vi "BonOMM-SAOMM.vi"() -> ()   [LabVIEW 2019] (continued)
                                n1114 = Insert Into Array(array=w4646, index=5, new element=w4645) -> (w4643:string[])
                                }
                                n1115 = local write "loaded_lib"(w4636) -> ()
                                n1116 = local write "Librairie des objets"(w4637) -> ()
                                n1117 = local write "Librairie complète"(w4637) -> ()
                              }
                            }
                          }
                          frame True {
                          }
                        }
                      }
                      frame "scp_Charger une libraire d'objets" {
                        # "Chemin à confirmer,\nvoir avec Mr Turbide ..."
                        # "Gestion du menu en développement ..."
                        n1118 = local read "path_libdir"() -> (w4657:path)
                        n1119 = File Dialog(6:"*.txt" ("pattern"), 7:"Sélectionner la libraire désirée ..." ("prompt"), 11:w4657) -> (0:w4658:errorcluster, 2:w4662:bool, 3:w4659:path)  [unwired: 4 in, 1 out]
                        n1120 = Unbundle(w4658) -> ()  [unwired: 3 out]
                        n1121 = case shown="Vrai" w4662 {
                          tunnel: w4659 -> [_ w4668]
                          frame False {
                          }
                          frame True {
                            n1122 = local write "loaded_lib"(w4668) -> ()
                            n1123 = local read "LST"() -> (w4665:dbl)
                            n1124 = call "Read_obs_files.vi"("Path"=w4668) -> ("Output Table"=w4673:string[][])  [unwired: 1 out]
                            n1125 = Strip Path(path=w4668) -> (stripped path=w4667:path)  [unwired: 1 out]
                            n1126 = for {
                              tunnel: w4673 -> [w4679] mode=indexing
                              tunnel: w4665 -> [w4680]
                              tunnel: [w4676] -> w4664 mode=indexing
                              n1127 = Index Array(array=w4679, index #1=2 ("index"), index #2=3 ("index")) -> (element #1=w4682:string, element #2=w4681:string)
                              n1128 = call "Airmass.vi"("temps sidéral"=w4680, "DEC"=w4681, "RA"=w4682) -> ("airmass"=w4677:dbl)
                              n1129 = Number To Fractional String(number=w4677, precision (6)=i16 2) -> (F-format string=w4678:string)  [unwired: 2 in]
                              n1130 = Insert Into Array(array=w4679, index=5, new element=w4678) -> (w4676:string[])
                            }
                            n1131 = Path To String(path=w4667) -> (string=w4669:string)
                            n1132 = local write "Librairie des objets"(w4664) -> ()
                            n1133 = control-ref of="TERMINAL"() -> (w4666:refnum<vi>)
                            n1134 = control-ref of="Indicateur d'état"() -> (w4663:refnum<vi>)
                            n1135 = Concatenate Strings("Chargement de la librairie \"", w4669, "\"") -> (w4672:string)
                            n1136 = call "TERMINAL.vi"("Indicateur Refnum"=w4663, "Terminal Refnum"=w4666, "Indicateur d'état"=w4672) -> ()
                          }
                        }
                      }
                      frame "scp_Modifier la liste des filtres" {
                        n1137 = call "ChoixFiltres.vi"("Ordre des filtres Avant"="Tableau des filtres") -> ("Ordre des filtres Après"=w4685:string[])
                        n1138 = local write "Tableau des filtres"(w4685) -> ()
                      }
                      frame "scp_Calibration du foyer automatique" {
                        # "À refaire avec le nouveau détecteur ..."
                      }
                      frame "scp_Calibration du champ" {
                        n1139 = local read "CentreTel X"() -> (w4690:dbl)
                        n1140 = local read "CentreTel Y"() -> (w4689:dbl)
                        n1141 = local read "Reference X"() -> (w4688:dbl)
                        n1142 = local read "Reference Y"() -> (w4687:dbl)
                        n1143 = local read "TableAstrom"() -> (w4692:T4)
                        n1144 = call "Starast.vi"("Ry"=w4687, "Rx"=w4688, "Centre Y"=w4689, "Centre X"=w4690, "Table Astrometry IN"=w4692) -> ("Table Astrometry OUT"=w4691:T4)  [unwired: 6 in]
                        n1145 = local write "TableAstrom"(w4691) -> ()
                      }
                    }
                  }
                  frame "main_Télescope" {
                    n1146 = case shown="\"tel_Test signal vers TCS\"" w4693 {
                      frame Default {
                      }
                      frame "tel_Synchroniser la coupole" {
                        n1147 = stacked-sequence {
                          frame #0 {
                            n1148 = control-ref of="TERMINAL"() -> (w4696:refnum<vi>)
                            n1149 = control-ref of="Indicateur d'état"() -> (w4695:refnum<vi>)
                            n1150 = call "TERMINAL.vi"("Indicateur Refnum"=w4695, "Terminal Refnum"=w4696, "Indicateur d'état"="Synchronisation de la coupole sur la position du télescope") -> ()
                          }
                          frame #1 {
                            # "Synchronise la coupole a la \nposition du télescope"
                            n1151 = control-ref of="TCS actif"() -> (w4697:refnum<vi>)
                            n1152 = local read "TCS VRN"() -> (w4704:refnum<visa-resource-name>)
                            n1153 = Build Array(0.0 ("string1")) -> (w4702:dbl[])
                            n1154 = call "EXCOM-CMD.vi"("VRN IN"=w4704, "Bool Refnum"=w4697, "Commande #"=2, "Args"=w4702) -> ("VRN OUT"=w4700:refnum<visa-resource-name>, "OK Done"=w4699:bool, "Error OUT"=w4698:errorcluster)  [unwired: 9 in]
                            n1155 = local write "TCS Error"(w4698) -> ()
                            n1156 = local write "TCS VRN"(w4700) -> ()
                            n1157 = case shown="Faux" w4699 {
                              frame False {
                                n1158 = One Button Dialog(message="ATTENTION!!\nLa commande de synchronisation de la coupole a échouée.\nVérifiez la communication avec TCS et recommencez.", button name ("OK")="OK" ("nom du bouton (\"OK\")")) -> ()  [unwired: 1 out]
                              }
                              frame True {
                              }
                            }
                          }
                        }
                      }
                      frame "tel_Synchroniser les horloges" {
                        n1159 = stacked-sequence {
                          seq-local: [w4710 _ _ _] -> [_ _ _ w4728]
                          frame #0 {
                            n1160 = local read "Epoch Tel"() -> (w4710:dbl)
                          }
                          frame #1 {
                            # "Initialise TCS"
                            n1161 = call "GetUTC.vi"() -> ("UTC_fractional"=w4720:dbl, "Day"=w4719:dbl, "Month"=w4718:dbl, "Year"=w4717:dbl, "DST?"=→"DST?":bool)  [unwired: 4 out]
                            n1162 = control-ref of="TCS actif"() -> (w4711:refnum<vi>)
                            n1163 = local read "TCS VRN"() -> (w4722:refnum<visa-resource-name>)
                            n1164 = Build Array(w4717, w4718, w4719, w4720) -> (w4716:dbl[])
                            n1165 = call "EXCOM-CMD.vi"("VRN IN"=w4722, "Bool Refnum"=w4711, "Commande #"=1, "Args"=w4716) -> ("VRN OUT"=w4715:refnum<visa-resource-name>, "OK Done"=w4714:bool, "Error OUT"=w4713:errorcluster)  [unwired: 9 in]
                            n1166 = local write "TCS Error"(w4713) -> ()
                            n1167 = local write "TCS VRN"(w4715) -> ()
                            n1168 = case shown="Vrai" w4714 {
                              frame False {
                                n1169 = One Button Dialog(message="ATTENTION!!\nLa commande INITIALISE TCS\na échoué.\nVérifiez TCS.", button name ("OK")="OK" ("nom du bouton (\"OK\")")) -> ()  [unwired: 1 out]
                              }
                              frame True {
                                n1170 = Wait (ms)(milliseconds to wait=u32 10 ("attente (ms)")) -> ()  [unwired: 1 out]
                              }
                            }
                          }
                          frame #2 {
                            n1171 = Wait (ms)(milliseconds to wait=u32 250) -> ()  [unwired: 1 out]
                          }
                          frame #3 {
                            n1172 = control-ref of="TCS actif"() -> (w4727:refnum<vi>)
                            n1173 = local read "TCS VRN"() -> (w4730:refnum<visa-resource-name>)
                            n1174 = Build Array(w4728) -> (w4733:dbl[])
                            n1175 = call "EXCOM-CMD.vi"("VRN IN"=w4730, "Bool Refnum"=w4727, "Commande #"=22, "Args"=w4733) -> ("VRN OUT"=w4731:refnum<visa-resource-name>, "Error OUT"=w4729:errorcluster)  [unwired: 9 in, 1 out]
                            n1176 = local write "TCS VRN"(w4731) -> ()
                            n1177 = local write "TCS Error"(w4729) -> ()
                          }
                        }
                        n1178 = control-ref of="TERMINAL"() -> (w4709:refnum<vi>)
                        n1179 = control-ref of="Indicateur d'état"() -> (w4708:refnum<vi>)
                        n1180 = call "TERMINAL.vi"("Indicateur Refnum"=w4708, "Terminal Refnum"=w4709, "Indicateur d'état"="Commande d'initialisation de TCS") -> ()
                      }
                      frame "tel_Modifier la vitesse du télescope" {
                        # "Changer la vitesse"
                        n1181 = control-ref of="TCS actif"() -> (w4734:refnum<vi>)
                        n1182 = local read "TCS VRN"() -> (w4738:refnum<visa-resource-name>)
                        n1183 = local read "TCS Error"() -> (w4736:errorcluster)
                        n1184 = control-ref of="TERMINAL"() -> (w4741:refnum<vi>)
                        n1185 = control-ref of="Indicateur d'état"() -> (w4742:refnum<vi>)
                        n1186 = call "Set speed.vi"("VRN IN"=w4738, "Bool Refnum"=w4734, "error IN"=w4736) -> ("VRN OUT"=w4737:refnum<visa-resource-name>, "OK Done"=w4739:bool, "error out"=w4735:errorcluster)  [unwired: 10 in]
                        n1187 = local write "TCS VRN"(w4737) -> ()
                        n1188 = local write "TCS Error"(w4735) -> ()
                        n1189 = call "TERMINAL.vi"("Indicateur Refnum"=w4742, "Terminal Refnum"=w4741, "Indicateur d'état"="Commande de changement des vitesse de TCS") -> ()
                        n1190 = case shown="Faux" w4739 {
                          frame False {
                            n1191 = One Button Dialog(message="ATTENTION!!\nLa commande CHANGER VITESSE a échoué.\nVérifiez TCS.", button name ("OK")="OK" ("nom du bouton (\"OK\")")) -> ()  [unwired: 1 out]
                          }
                          frame True {
                          }
                        }
                      }
                      frame "tel_Modifier la vitesse de guidage" {
                        n1192 = local read "RateRA"() -> (w4749:dbl)
                        n1193 = expression code="1000/x"(w4749) -> (w4748:dbl)
                        n1194 = call "GuideRate.vi"("Guide Rate"=w4748) -> ("Guide Rate out"=w4746:dbl)  [unwired: 14 in]
                        n1195 = Build Array(w4746) -> (w4747:dbl[])
                        n1196 = expression code="1000/x"(w4746) -> (w4745:dbl)
                        n1197 = control-ref of="TCS actif"() -> (w4752:refnum<vi>)
                        n1198 = local read "TCS VRN"() -> (w4753:refnum<visa-resource-name>)
                        n1199 = call "EXCOM-CMD.vi"("VRN IN"=w4753, "Bool Refnum"=w4752, "Commande #"=15, "Args"=w4747) -> ("VRN OUT"=w4754:refnum<visa-resource-name>, "Error OUT"=w4750:errorcluster)  [unwired: 9 in, 1 out]
                        n1200 = local write "RateDEC"(w4745) -> ()
                        n1201 = local write "RateRA"(w4745) -> ()
                        n1202 = local write "TCS Error"(w4750) -> ()
                        n1203 = local write "TCS VRN"(w4754) -> ()
                      }
                      frame "tel_Modifier l'époque d'affichage" {
                        # "Ne change pas l'équinoxe de TCS mais seulement l'affichage pour BonOMM"
                        n1204 = local read "Epoch Tel"() -> (w4756:dbl)
                        n1205 = local read "AnnéeRL"() -> (w4757:dbl)
                        n1206 = call "Set_epoch.vi"("AnnéeRL"=w4757, "EPOCH_AFF"=w4756) -> ("EPOCH_OUT"=w4755:dbl)
                        n1207 = local write "dflt-EQX"(w4755) -> ()
                        n1208 = disable-structure shown="Disabled" {
                          disable-tunnel: w4755 -> [w4758 _]
                          frame Disabled {
                            n1209 = control-ref of="TCS actif"() -> (w4759:refnum<vi>)
                            n1210 = local read "TCS VRN"() -> (w4765:refnum<visa-resource-name>)
                            n1211 = Build Array(w4758) -> (w4760:dbl[])
                            n1212 = call "EXCOM-CMD.vi"("VRN IN"=w4765, "Bool Refnum"=w4759, "Commande #"=22 ("NombredArguments"), "Args"=w4760) -> ("VRN OUT"=w4763:refnum<visa-resource-name>, "OK Done"=w4761:bool, "Error OUT"=w4762:errorcluster)  [unwired: 9 in]
                            n1213 = local write "TCS Error"(w4762) -> ()
                            n1214 = local write "TCS VRN"(w4763) -> ()
                            n1215 = case shown="Faux" w4761 {
                              frame False {
                                n1216 = One Button Dialog(message="Erreur lors du chargement de la nouvelle époque d'affichage.\nVérifier la communication avec TCS et recommencez.") -> ()  [unwired: 1 in, 1 out]
                              }
                              frame True {
                              }
                            }
                          }
                          frame Enabled {
                          }
                        }
                      }
                      frame "tel_Test signal vers TCS" {
                        n1217 = call "Test_telecommande.vi"() -> ()  [unwired: 1 in]
                      }
                      frame "tel_Reconnexion" {
                        n1218 = One Button Dialog(message="Devrait reconnecter TCS ...") -> ()  [unwired: 1 in, 1 out]
                      }
                    }
                  }
                  frame "main_Secondaire Actif" {
                    n1219 = case shown="\"hex_Déplacement manuel\"" w4768 {
                      frame Default {
                      }
                      frame "hex_Commander l'hexapode" {
                        n1220 = flat-sequence {
                          frame #0 {
                            "HexaSpam" <- TRUE ("HexaSpam")
                          }
                          frame #1 {
                            # "Attention, erreur d'époque possible ..."
                            n1221 = disable-structure shown="Disabled" {
                              frame Disabled {
                                # "Rafraichi la position de l'hexapode 2x par seconde"
                                n1222 = local read "Hexapod VRN"() -> (w4786:refnum<visa-resource-name>)
                                n1223 = local read "MessageType"() -> (w4787:cluster{string[], u32[]})
                                n1224 = local read "PrAMS VRN"() -> (w4789:refnum<visa-resource-name>)
                                n1225 = control-ref of="HexX"() -> (w4772:refnum<vi>)
                                n1226 = control-ref of="HexY"() -> (w4773:refnum<vi>)
                                n1227 = control-ref of="HexZ"() -> (w4774:refnum<vi>)
                                n1228 = control-ref of="HexU"() -> (w4775:refnum<vi>)
                                n1229 = control-ref of="HexV"() -> (w4776:refnum<vi>)
                                n1230 = local read "Signature"() -> (w4788:u32)
                                n1231 = Bundle("PrAMS VRN"=w4789, "Signature"=w4788, "MessageType"=w4787, "Hexapod VRN"=w4786) -> (w4785:T28)  [unwired: 1 in]
                                n1232 = Bundle("HexX"=w4772, "HexY"=w4773, "HexZ"=w4774, "HexU"=w4775, "HexV"=w4776) -> (w4771:T29)  [unwired: 1 in]
                                n1233 = control-ref of="Angle Hor."() -> (w4779:refnum<vi>)
                                n1234 = control-ref of="DEC Tel"() -> (w4778:refnum<vi>)
                                n1235 = control-ref of="PrAMS-ACK"() -> (w4781:refnum<vi>)
                                n1236 = control-ref of="Hexapod-ACK"() -> (w4783:refnum<vi>)
                                n1237 = control-ref of="Epoch Tel"() -> (w4770:refnum<vi>)
                                n1238 = control-ref of="PrAMS actif"() -> (w4784:refnum<vi>)
                                n1239 = control-ref of="HexaCons actif"() -> (w4782:refnum<vi>)
                                n1240 = Bundle("Angle Hor."=w4779, "DEC Tel"=w4778, "Epoch Tel"=w4770) -> (w4777:T30)  [unwired: 1 in]
                                n1241 = flat-sequence {
                                tunnel: w4785 -> [w4793]
                                tunnel: w4780 -> [w4792]
                                tunnel: w4777 -> [w4791]
                                tunnel: w4771 -> [w4790]
                                frame #0 {
                                n1242 = call "Hexapod-Console.vi"("CommCluster"=w4793, "ReferenceCluster"=w4792, "TelescopeCLuster"=w4791, "HexapodCluster"=w4790) -> ()  [unwired: 12 in]
                                }
                                frame #1 {
                                n1243 = local write "HexaSpam"(FALSE ("HexaSpam")) -> ()
                                }
                                }
                                n1244 = while {
                                stop <- w4796 continue-if-true
                                n1245 = Wait (ms)(milliseconds to wait=u32 500) -> ()  [unwired: 1 out]
                                n1246 = local read "HexaSpam"() -> (w4796:bool)
                                n1247 = property on="HexapodRefresh" class="Bool (strict)"("Val(Sgnl)"=TRUE ("Value (Signaling)")) -> ()  [unwired: 2 in, 2 out]
                                }
                                n1248 = Bundle("PrAMS actif"=w4784, "PrAMS-ACK"=w4781, "HexaCons actif"=w4782, "Hexapod-ACK"=w4783) -> (w4780:T31)  [unwired: 1 in]
                              }
                              frame Enabled {
                                n1249 = One Button Dialog(message="Fonction en développement ...\n\nUtilisez plutôt \"déplacement manuel\"") -> ()  [unwired: 1 in, 1 out]
                              }
                            }
                          }
                        }
                      }
                      frame "hex_Paramètres d'asservissement" {
                        # "Ici, on voudra probablement :\n  - Modifier la fréquence du filtre\n  - Modifier le nombre d'image prises en compte\n  - Modifier le coefficient d'aggressivité\n  - Modifier l'affichage de l'historique"
                        n1250 = One Button Dialog(message="Interaction usagé à définir ...") -> ()  [unwired: 1 in, 1 out]
                      }
                      frame "hex_Panneau de offset" {
                        n1251 = flat-sequence {
                          tunnel: [w4806] -> w4800
                          tunnel: w4800 -> [w4813]
                          frame #0 {
                            n1252 = local read "Mode"() -> (w4801:u16)
                            n1253 = case shown="0" w4801 {
                              frame Default {
                              }
                              frame 0 {
                                n1254 = One Button Dialog(message="Il semble que le système ne soit pas en mode \"collimation\".\n\nPour que les valeurs de offsets demandés prennent effets, il\nest essentiel que le système soit en mode \"collimation\" ou \ntout autre mode utilisant l'hexapode.\n\nPour lancer le mode collimation, lancer d'abord l'exposition\nde la caméra de guidage puis sélectionné \"collimation\".\n\nL'application permettant de charger les offsets d'hexapode\nsera tout de même lancé, mais l'effet ne sera appliqué que\nlors du lancement d'un des modes utilisant l'hexapode.", button name ("OK")="J'ai lu et compris, merci.") -> ()  [unwired: 1 out]
                              }
                            }
                          }
                          frame #1 {
                            n1255 = local write "QueryingHexapod"(TRUE ("Value (Signaling)")) -> ()
                            n1256 = property on="HexapodRefresh" class="Bool (strict)"("Val(Sgnl)"=TRUE ("Value (Signaling)")) -> ()  [unwired: 2 in, 2 out]
                          }
                          frame #2 {
                            n1257 = while {
                              tunnel: [w4807] -> w4806
                              i -> [w4811]
                              stop <- w4810 stop-if-true
                              n1258 = local read "QueryingHexapod"() -> (w4807:bool)
                              n1259 = Not(x=w4807) -> (.not. x?=w4809:bool)
                              n1260 = Wait (ms)(milliseconds to wait=u32 100) -> ()  [unwired: 1 out]
                              n1261 = call "Max-iteration.vi"("i max"=50, "i act"=w4811, "Valeur entrante"=w4809) -> ("break ?"=w4810:bool)
                            }
                          }
                          frame #3 {
                            n1262 = case shown="Faux" w4813 {
                              frame False {
                                n1263 = control-ref of="Hexapod-ACK"() -> (w4816:refnum<vi>)
                                n1264 = control-ref of="Offset X"() -> (w4820:refnum<vi>)
                                n1265 = control-ref of="Offset Y"() -> (w4821:refnum<vi>)
                                n1266 = control-ref of="Offset Z"() -> (w4822:refnum<vi>)
                                n1267 = control-ref of="Offset U"() -> (w4823:refnum<vi>)
                                n1268 = control-ref of="Offset V"() -> (w4824:refnum<vi>)
                                n1269 = local read "Hexapod VRN"() -> (w4817:refnum<visa-resource-name>)
                                n1270 = local read "MessageType"() -> (w4814:cluster{string[], u32[]})
                                n1271 = control-ref of="HexaCons actif"() -> (w4815:refnum<vi>)
                                n1272 = Bundle("Offset X"=w4820, "Offset Y"=w4821, "Offset Z"=w4822, "Offset U"=w4823, "Offset V"=w4824) -> (w4819:T32)  [unwired: 1 in]
                                n1273 = call "TEST-SAOMM-OffsetGUI.vi"("Hexapod VRN"=w4817, "Active Refnum"=w4815, "PrAMS-ACK"=w4816, "output cluster"=w4819, "MessageType"=w4814) -> ("Error"=w4818:bool)  [unwired: 10 in]
                                n1274 = case shown="Vrai" w4818 {
                                frame False {
                                }
                                frame True {
                                n1275 = One Button Dialog(message="Erreur lors de l'envoi\ndes valeurs de l'offset.") -> ()  [unwired: 1 in, 1 out]
                                }
                                }
                              }
                              frame True {
                                n1276 = One Button Dialog(message="Les valeurs de offsets n'ont pu être lu !?!\nVérifiez la connexion à \"hexapode-console\"") -> ()  [unwired: 1 in, 1 out]
                              }
                            }
                          }
                        }
                      }
                      frame "hex_Déplacement manuel" {
                        n1277 = flat-sequence {
                          tunnel: [w4830] -> w4827
                          tunnel: w4827 -> [w4837]
                          frame #0 {
                            n1278 = local write "QueryingHexapod"(TRUE ("Value (Signaling)")) -> ()
                            n1279 = property on="HexapodRefresh" class="Bool (strict)"("Val(Sgnl)"=TRUE ("Value (Signaling)")) -> ()  [unwired: 2 in, 2 out]
                          }
                          frame #1 {
                            n1280 = while {
                              tunnel: [w4831] -> w4830
                              i -> [w4835]
                              stop <- w4834 stop-if-true
                              n1281 = local read "QueryingHexapod"() -> (w4831:bool)
                              n1282 = Not(x=w4831) -> (.not. x?=w4833:bool)
                              n1283 = Wait (ms)(milliseconds to wait=u32 100) -> ()  [unwired: 1 out]
                              n1284 = call "Max-iteration.vi"("i max"=50, "i act"=w4835, "Valeur entrante"=w4833) -> ("break ?"=w4834:bool)
                            }
                          }
                          frame #2 {
                            n1285 = case shown="Faux" w4837 {
                              frame False {
                                n1286 = control-ref of="Hexapod-ACK"() -> (w4840:refnum<vi>)
                                n1287 = control-ref of="HexX"() -> (w4844:refnum<vi>)
                                n1288 = control-ref of="HexY"() -> (w4845:refnum<vi>)
                                n1289 = control-ref of="HexZ"() -> (w4846:refnum<vi>)
                                n1290 = control-ref of="HexU"() -> (w4847:refnum<vi>)
                                n1291 = control-ref of="HexV"() -> (w4848:refnum<vi>)
                                n1292 = local read "Hexapod VRN"() -> (w4841:refnum<visa-resource-name>)
                                n1293 = local read "MessageType"() -> (w4838:cluster{string[], u32[]})
                                n1294 = control-ref of="HexaCons actif"() -> (w4839:refnum<vi>)
                                n1295 = Bundle("HexX"=w4844, "HexY"=w4845, "HexZ"=w4846, "HexU"=w4847, "HexV"=w4848) -> (w4843:T29)  [unwired: 1 in]
                                n1296 = call "TEST-SAOMM-PositionGUI.vi"("Hexapod VRN"=w4841, "Active Refnum"=w4839, "PrAMS-ACK"=w4840, "output cluster"=w4843, "MessageType"=w4838) -> ("Error"=w4842:bool)  [unwired: 10 in]
                                n1297 = case shown="Vrai" w4842 {
                                frame False {
                                }
                                frame True {
                                n1298 = One Button Dialog(message="Erreur lors de l'envoi\ndes valeurs de l'offset.") -> ()  [unwired: 1 in, 1 out]
                                }
                                }
                              }
                              frame True {
                                n1299 = One Button Dialog(message="Les valeurs de offsets n'ont pu être lu !?!\nVérifiez la connexion à \"hexapode-console\"") -> ()  [unwired: 1 in, 1 out]
                              }
                            }
                          }
                        }
                      }
                      frame "hex_Remise à zéro" {
                        n1300 = control-ref of="Hexapod-ACK"() -> (w4859:refnum<vi>)
                        n1301 = local read "Hexapod VRN"() -> (w4858:refnum<visa-resource-name>)
                        n1302 = local read "MessageType"() -> (w4855:cluster{string[], u32[]})
                        n1303 = control-ref of="HexaCons actif"() -> (w4860:refnum<vi>)
                        n1304 = local read "HexU"() -> (w4854:dbl)
                        n1305 = local read "HexV"() -> (w4853:dbl)
                        n1306 = local read "Signature"() -> (w4857:u32)
                        n1307 = local read "PrAMS Error"() -> (w4856:errorcluster)
                        n1308 = call "SAOMM-RaZ.vi"("PRAMMS-COMM IN"=w4858, "Active Refnum"=w4860, "PrAMS-ACK"=w4859, "Signature"=w4857, "Error IN"=w4856, "MessageType"=w4855, "Position U"=w4854, "Position V"=w4853) -> ("PRAMMS-COMM OUT"=w4852:refnum<visa-resource-name>, "Error OUT"=w4851:errorcluster)  [unwired: 6 in]
                        n1309 = local write "Hexapod VRN"(w4852) -> ()
                        n1310 = local write "PrAMS Error"(w4851) -> ()
                      }
                    }
                  }
                  frame "main_Caméra de référence" {
                    n1311 = case shown="\"cam_Reconnexion\"" w4862 {
                      selector: w4862 -> [_ _ _ _ w4949 _]
                      tunnel: w4861 -> [_ _ _ _ _ _]
                      frame Default {
                      }
                      frame "cam_Enregistrer la prochaine image" {
                        n1312 = local write "SaveNextImage"(TRUE ("SaveNextImage")) -> ()
                      }
                      frame "cam_Modifier les paramètres" {
                        n1313 = flat-sequence {
                          tunnel: [w4903] -> w4870
                          tunnel: w4870 -> [w4916]
                          tunnel: [w4915] -> w4869
                          tunnel: [w4914] -> w4868
                          tunnel: [w4913] -> w4867
                          tunnel: [w4912] -> w4866
                          tunnel: [w4911] -> w4865
                          tunnel: [w4910] -> w4864
                          frame #0 {
                            n1314 = local write "QueryingPraMS"(TRUE ("Querying")) -> ()
                            n1315 = property on="FalconRefresh" class="Bool (strict)"("Val(Sgnl)"=TRUE ("Value (Signaling)")) -> ()  [unwired: 2 in, 2 out]
                          }
                          frame #1 {
                            n1316 = while {
                              tunnel: [w4905] -> w4903
                              i -> [w4909]
                              stop <- w4908 stop-if-true
                              n1317 = local read "QueryingPraMS"() -> (w4906:bool)
                              n1318 = Not(x=w4906) -> (.not. x?=w4905:bool)
                              n1319 = Wait Until Next ms Multiple(millisecond multiple=u32 50) -> ()  [unwired: 1 out]
                              n1320 = call "Max-iteration.vi"("i max"=100, "i act"=w4909, "Valeur entrante"=w4905) -> ("break ?"=w4908:bool)
                            }
                          }
                          frame #2 {
                            n1321 = case shown="Vrai" w4916 {
                              tunnel: [FALSE ("Apply Changes") w4933] -> w4915
                              tunnel: [u16 0 ("Gain_OUT") w4932] -> w4914
                              tunnel: [u16 0 ("Binning_OUT") w4931] -> w4913
                              tunnel: [0.0 ("FPS_OUT") w4930] -> w4912
                              tunnel: [u16 0 ("Cooling_OUT") w4927] -> w4911
                              tunnel: [0 ("Binning_OUT") w4924] -> w4910
                              frame False {
                                n1322 = One Button Dialog(message="Problème de communication avec Prams") -> ()  [unwired: 1 in, 1 out]
                              }
                              frame True {
                                n1323 = property on="ROIsurface" class="MDér (strict)"() -> ("Strings []"=w4925:string[])  [unwired: 2 in, 2 out]
                                n1324 = local read "ImageFPS"() -> (w4934:dbl)
                                n1325 = local read "FPGA Value"() -> (w4928:u16)
                                n1326 = local read "ROIsurface"() -> (w4926:i32)
                                n1327 = local read "EMGain"() -> (w4929:u16)
                                n1328 = local read "Binning"() -> (w4935:u16)
                                n1329 = call "CameraSettings.vi"("Région d'intérêt"=w4926, "ROIStrings"=w4925, "Gain EM"=w4929, "Refroidissement"=w4928, "Binning"=w4935, "FPS"=w4934) -> ("Apply Changes"=w4933:bool, "Cooling_OUT"=w4927:u16, "Gain_OUT"=w4932:u16, "Binning_OUT"=w4931:u16, "ROISize_OUT"=w4924:i32, "FPS_OUT"=w4930:dbl)  [unwired: 4 in]
                              }
                            }
                          }
                        }
                        n1330 = case shown="Vrai" w4869 {
                          tunnel: w4868 -> [_ w4884]
                          tunnel: w4867 -> [_ w4881]
                          tunnel: w4866 -> [_ w4877]
                          tunnel: w4865 -> [_ w4876]
                          tunnel: w4864 -> [_ w4872]
                          frame False {
                          }
                          frame True {
                            n1331 = flat-sequence {
                              tunnel: [w4890] -> w4885
                              tunnel: w4884 -> [w4890]
                              tunnel: [w4889] -> w4882
                              tunnel: w4881 -> [w4889]
                              tunnel: [w4888] -> w4878
                              tunnel: w4877 -> [w4888]
                              tunnel: w4876 -> [w4887]
                              tunnel: [w4886] -> w4873
                              tunnel: w4872 -> [w4886]
                              tunnel: w4885 -> [w4892]
                              tunnel: [w4894] -> w4883
                              tunnel: w4882 -> [w4894]
                              tunnel: [w4893] -> w4879
                              tunnel: w4878 -> [w4893]
                              tunnel: [w4891] -> w4874
                              tunnel: w4873 -> [w4891]
                              tunnel: w4883 -> [w4896]
                              tunnel: [w4897] -> w4880
                              tunnel: w4879 -> [w4897]
                              tunnel: [w4895] -> w4875
                              tunnel: w4874 -> [w4895]
                              tunnel: w4880 -> [w4899]
                              tunnel: w4875 -> [w4898]
                              tunnel: [w4898] -> w4871
                              tunnel: w4871 -> [w4900]
                              frame #0 {
                                n1332 = property on="FPGA Value" class="MDér (strict)"("Val(Sgnl)"=w4887) -> ()  [unwired: 2 in, 2 out]
                              }
                              frame #1 {
                                n1333 = property on="EMGain" class="NumNb (strict)"("Val(Sgnl)"=w4892) -> ()  [unwired: 2 in, 2 out]
                              }
                              frame #2 {
                                n1334 = property on="Binning" class="MDér (strict)"("Val(Sgnl)"=w4896) -> ()  [unwired: 2 in, 2 out]
                              }
                              frame #3 {
                                n1335 = property on="ImageFPS" class="NumNb (strict)"("Val(Sgnl)"=w4899) -> ()  [unwired: 2 in, 2 out]
                              }
                              frame #4 {
                                n1336 = property on="ROIsurface" class="MDér (strict)"("Val(Sgnl)"=w4900) -> ()  [unwired: 2 in, 2 out]
                              }
                            }
                          }
                        }
                      }
                      frame "cam_Modifier la région d'intérêt" {
                        n1337 = local read "ROIXOffset"() -> (w4946:u16)
                        n1338 = local read "ROIYOffset"() -> (w4945:u16)
                        n1339 = local read "ROIHeight"() -> (w4943:u16)
                        n1340 = local read "ROIWidth"() -> (w4944:u16)
                        n1341 = local read "ImgArray"() -> (w4941:u32[][])
                        n1342 = property on="ROIsurface" class="MDér (strict)"() -> ("Strings []"=w4947:string[])  [unwired: 2 in, 2 out]
                        n1343 = local read "ROISizes"() -> (w4942:u16[])
                        n1344 = call "ROISettings.vi"("ROISizes"=w4942, "SizeEnum"=w4947, "ImgArray"=w4941, "ROIHeight"=w4943, "ROIWidth"=w4944, "ROIYOffset"=w4945, "ROIXOffset"=w4946) -> ("ROIHeightOUT"=w4937:u16, "ROIWidthOUT"=w4938:u16, "ROIYOffsetOUT"=w4939:u16, "ROIXOffsetOUT"=w4940:u16, "SizesOUT"=w4936:i32)
                        n1345 = local write "ROIXOffset"(w4940) -> ()
                        n1346 = local write "ROIYOffset"(w4939) -> ()
                        n1347 = local write "ROIHeight"(w4937) -> ()
                        n1348 = local write "ROIWidth"(w4938) -> ()
                        n1349 = property on="ROIsurface" class="MDér (strict)"("Val(Sgnl)"=w4936) -> ()  [unwired: 2 in, 2 out]
                      }
                      frame "cam_Binning 1x1", "cam_Binning 2x2", "cam_Binning 4x4", "cam_Binning 5x5" {
                        n1350 = case shown="\"cam_Binning 5x5\"" w4949 {
                          tunnel: [u16 1 u16 1 u16 2 u16 4 u16 5] -> w4948
                          frame Default {
                          }
                          frame "cam_Binning 1x1" {
                          }
                          frame "cam_Binning 2x2" {
                          }
                          frame "cam_Binning 4x4" {
                          }
                          frame "cam_Binning 5x5" {
                          }
                        }
                        n1351 = property on="Binning" class="MDér (strict)"("Val(Sgnl)"=w4948) -> ()  [unwired: 2 in, 2 out]
                      }
                      frame "cam_Reconnexion" {
                        n1352 = One Button Dialog(message="Devrait reconnecter Prams ...") -> ()  [unwired: 1 in, 1 out]
                      }
                    }
                  }
                  frame "main_Tables de guidage" {
                    n1353 = case shown="\"tab_Commandes XYZ\"" w4956 {
                      frame Default {
                      }
                      frame "tab_Modifier les vitesses des tables" {
                        # "GUI pour modifier la vitesse des tales ..."
                        n1354 = local read "vitesse lente"() -> (w4962:dbl)
                        n1355 = local read "accelleration"() -> (w4961:dbl)
                        n1356 = local read "vitesse focus"() -> (w4958:dbl)
                        n1357 = local read "vitesse rapide"() -> (w4964:dbl)
                        n1358 = call "Set_table_speed.vi"("Z IN"=w4958, "Accel IN"=w4961, "Fast IN"=w4964, "slow IN"=w4962) -> ("Z OUT"=w4957:dbl, "Accel OUT"=w4959:dbl, "Fast OUT"=w4963:dbl, "slow OUT"=w4960:dbl)  [unwired: 4 in]
                        n1359 = local write "vitesse rapide"(w4963) -> ()
                        n1360 = local write "accelleration"(w4959) -> ()
                        n1361 = local write "vitesse focus"(w4957) -> ()
                        n1362 = local write "vitesse lente"(w4960) -> ()
                      }
                      frame "tab_Positions prédéfinies" {
                        n1363 = local read "Rangement X"() -> (w4974:dbl)
                        n1364 = local read "Rangement Y"() -> (w4975:dbl)
                        n1365 = local read "Rangement Z"() -> (w4973:dbl)
                        n1366 = local read "Calibration X"() -> (w4984:dbl)
                        n1367 = local read "Calibration Y"() -> (w4983:dbl)
                        n1368 = local read "Reference X"() -> (w4981:dbl)
                        n1369 = local read "Reference Y"() -> (w4980:dbl)
                        n1370 = local read "CentreTel X"() -> (w4978:dbl)
                        n1371 = local read "CentreTel Y"() -> (w4977:dbl)
                        n1372 = local read "Position X"() -> (w4972:dbl)
                        n1373 = local read "Position Y"() -> (w4971:dbl)
                        n1374 = Bundle("CentreTel X"=w4978, "CentreTel Y"=w4977) -> (w4976:cluster{"CentreTel X":dbl, "CentreTel Y":dbl})  [unwired: 1 in]
                        n1375 = Bundle("Reference X"=w4981, "Reference Y"=w4980) -> (w4979:cluster{"Reference X":dbl, "Reference Y":dbl})  [unwired: 1 in]
                        n1376 = Bundle("Calibration X"=w4984, "Calibration Y"=w4983) -> (w4982:T33)  [unwired: 1 in]
                        n1377 = Bundle("Rangement X"=w4974, "Rangement Y"=w4975, "Rangement Z"=w4973) -> (w4968:T34)  [unwired: 1 in]
                        n1378 = call "Set_predefined_table_positions.vi"("Calibration IN"=w4982, "Position Y"=w4971, "Position X"=w4972, "Reference IN"=w4979, "Centre IN"=w4976, "Park IN"=w4968) -> ("Calibration OUT"=w4969:T35, "Reference OUT"=w4965:cluster{"Reference Y":dbl, "Reference X":dbl}, "Centre OUT"=w4966:cluster{"Centre Y":dbl, "Centre X":dbl}, "Accept?"=w4970:bool, "Park OUT"=w4967:T36)  [unwired: 5 in]
                        n1379 = case shown="Vrai" w4970 {
                          tunnel: w4969 -> [_ w4997]
                          tunnel: w4967 -> [_ w4994]
                          tunnel: w4966 -> [_ w4990]
                          tunnel: w4965 -> [_ w4987]
                          frame False {
                          }
                          frame True {
                            n1380 = Unbundle(w4997) -> ("Calibration Y"=w4996:dbl, "Calibration X"=w4995:dbl)
                            n1381 = Unbundle(w4990) -> ("Centre Y"=w4989:dbl, "Centre X"=w4988:dbl)
                            n1382 = Unbundle(w4987) -> ("Reference Y"=w4986:dbl, "Reference X"=w4985:dbl)
                            n1383 = Unbundle(w4994) -> ("Range Y"=w4993:dbl, "Range X"=w4992:dbl, "Range Z"=w4991:dbl)
                            n1384 = local write "Rangement X"(w4993) -> ()
                            n1385 = local write "Rangement Y"(w4992) -> ()
                            n1386 = local write "Rangement Z"(w4991) -> ()
                            n1387 = local write "Calibration X"(w4996) -> ()
                            n1388 = local write "Calibration Y"(w4995) -> ()
                            n1389 = local write "Reference X"(w4986) -> ()
                            n1390 = local write "Reference Y"(w4985) -> ()
                            n1391 = local write "CentreTel X"(w4989) -> ()
                            n1392 = local write "CentreTel Y"(w4988) -> ()
                          }
                        }
                      }
                      frame "tab_Commandes XYZ" {
                        n1393 = local read "MovingZ"() -> (w5000:bool)
                        n1394 = local read "MovingXY"() -> (w4999:bool)
                        n1395 = Or(x=w5000, y=w4999) -> (x .or. y?=w4998:bool)
                        n1396 = case shown="Faux" w4998 {
                          frame False {
                            n1397 = control-ref of="Table actif"() -> (w5004:refnum<vi>)
                            n1398 = control-ref of="BrasPesto"() -> (w5002:refnum<vi>)
                            n1399 = control-ref of="LimXPesto"() -> (w5001:refnum<vi>)
                            n1400 = control-ref of="Table VRN"() -> (w5006:refnum<vi>)
                            n1401 = control-ref of="Table Error"() -> (w5005:refnum<vi>)
                            n1402 = control-ref of="Cible X"() -> (w5009:refnum<vi>)
                            n1403 = control-ref of="Cible Y"() -> (w5010:refnum<vi>)
                            n1404 = control-ref of="Cible Z"() -> (w5008:refnum<vi>)
                            n1405 = local read "Position X"() -> (w5013:dbl)
                            n1406 = local read "Position Y"() -> (w5012:dbl)
                            n1407 = local read "Position Z"() -> (w5011:dbl)
                            n1408 = Bundle("Cible X"=w5009, "Cible Y"=w5010, "Cible Z"=w5008) -> (w5007:T37)  [unwired: 1 in]
                            n1409 = Bundle("Table VRN"=w5006, "Table Error"=w5005, "Table actif"=w5004, "BrasPesto"=w5002, "LimXPesto"=w5001) -> (w5003:T38)  [unwired: 1 in]
                            n1410 = call "CommandesXYZ.vi"("Structure-Communications"=w5003, "Structure-Cibles"=w5007, "Position X"=w5013, "Position Y"=w5012, "Position Z"=w5011) -> ()  [unwired: 11 in]
                          }
                          frame True {
                            n1411 = One Button Dialog(message="Les tables de translation semblent déjà être\nen mouvement, assurez-vous qu'elles sont arrêtées\navant de lancer le mode \"XYZ\".") -> ()  [unwired: 1 in, 1 out]
                          }
                        }
                      }
                      frame "tab_Modifier les paramètres" {
                        # "ClickJOG est en minute d'arc ..."
                        n1412 = local read "ClickJOG"() -> (w5018:dbl)
                        n1413 = expression code="x*60.0"(w5018) -> (w5017:dbl)
                        n1414 = call "Set-Jog-Params.vi"("clic IN"=w5017) -> ("clic OUT"=w5016:dbl)  [unwired: 14 in]
                        n1415 = expression code="x/60.0"(w5016) -> (w5015:dbl)
                        n1416 = local write "ClickJOG"(w5015) -> ()
                      }
                      frame "Reconnexion" {
                      }
                    }
                  }
                  frame "main_Roue à filtres" {
                    n1417 = case shown="\"raf_Reconnexion\"" w5019 {
                      selector: w5019 -> [w5025 _ _]
                      frame Default {
                        w5023 = "@@"
                        # "hmm, à compléter ...\n\n  - Cocher le filtre en place\n  - Commencer par rafraichir\n  - Si déconnecté, ne pas permettre un déplacement de la roue ..."
                        n1418 = Search/Split String(string=w5025, search string/char (-)=w5023) -> (match + rest of string=w5024:string)  [unwired: 1 in, 2 out]
                        n1419 = String Length(string=w5023) -> (length=w5022:i32)
                        n1420 = String Subset(string=w5024, offset (0)=w5022) -> (substring=w5021:string)  [unwired: 1 in]
                        n1421 = Decimal String To Number(string=w5021) -> (number=w5020:i32)  [unwired: 2 in, 1 out]
                        n1422 = Greater Or Equal To 0?(x=w5020) -> (x >= 0?=w5026:bool)
                        n1423 = case shown="Vrai" w5026 {
                          tunnel: w5020 -> [_ w5038]
                          frame False {
                          }
                          frame True {
                            n1424 = Replace Array Subset(array=bool[] [FALSE, FALSE, FALSE, FALSE, FALSE, FALSE], new element=TRUE ("new element/subarray"), index=w5038) -> (w5032:bool[])
                            n1425 = property on="ChoixFiltre" class="Clust (strict)"() -> ("Value"=w5035:T12)  [unwired: 2 in, 2 out]
                            n1426 = Index Array(array=w5032) -> (element #1=w5033:bool, element #2=w5031:bool, element #3=w5030:bool, element #4=w5029:bool, element #5=w5028:bool, element #6=w5027:bool)  [unwired: 6 in]
                            n1427 = Bundle(cluster=w5035, "filtre #1"=w5033, "filtre #2"=w5031, "filtre #3"=w5030, "filtre #4"=w5029, "filtre #5"=w5028, "filtre #6"=w5027) -> (w5034:T12)
                            n1428 = property on="ChoixFiltre" class="Clust (strict)"("Val(Sgnl)"=w5034) -> ()  [unwired: 2 in, 2 out]
                          }
                        }
                      }
                      frame "raf_Modifier la liste des filtres" {
                        n1429 = flat-sequence {
                          frame #0 {
                            n1430 = local write "HautDroit"(T11."Périphérique" ("HautDroit")) -> ()
                          }
                          frame #1 {
                            n1431 = property on="change_filtre_liste" class="Bool (strict)"("Val(Sgnl)"=TRUE) -> ()  [unwired: 2 in, 2 out]
                          }
                        }
                      }
                      frame "raf_Reconnexion" {
                        n1432 = flat-sequence {
                          frame #0 {
                            w5042 = u16 0 items=["Roue à Filtres (BonOMM)", "Roue à Filtres (PANO-II)", "Foyer ST-133", "Lampes d'étalonnage", "Options des périphériques"] ("Périphérique")
                            n1433 = local write "HautDroit"(T11."Périphérique" ("HautDroit")) -> ()
                            n1434 = local write "Périphérique"(w5042) -> ()
                          }
                          frame #1 {
                            n1435 = property on="reconnect" class="Bool (strict)"("Val(Sgnl)"=TRUE ("Value (Signaling)")) -> ()  [unwired: 2 in, 2 out]
                          }
                        }
                      }
                    }
                  }
                  frame "main_FA" {
                    n1436 = case shown="\"fa_Mode Guidage et Dither\"" w5044 {
                      selector: w5044 -> [_ w5045]
                      frame "False", Default {
                      }
                      frame "fa_Mode Guidage et Dither" {
                        n1437 = case shown="Faux" "Mode Guidage et Dither" {
                          tunnel: w5045 -> [w5047 w5050]
                          frame False {
                            w5049 = TRUE ("Mode Guidage et Dither")
                            n1438 = Current VI's Menubar() -> (w5048:refnum<k9>)
                            n1439 = Set Menu Item Info(6:w5049, 7:w5047, 11:w5048) -> ()  [unwired: 4 in, 2 out]
                            n1440 = local write "Mode Guidage et Dither"(w5049) -> ()
                          }
                          frame True {
                            n1441 = Current VI's Menubar() -> (w5052:refnum<k9>)
                            n1442 = Set Menu Item Info(6:FALSE ("checked"), 7:w5050, 11:w5052) -> ()  [unwired: 4 in, 2 out]
                            n1443 = local write "Mode Guidage et Dither"(FALSE ("Mode Guidage et Dither")) -> ()
                          }
                        }
                      }
                    }
                  }
                }
              }
              event Key Down {
                n1444 = event-data() -> ("Char"=w5054:i16, "ScanCode"=w5055:i16)  [unwired: 1 in, 7 out]
                n1445 = case shown="101" w5054 {
                  tunnel: w5055 -> [_ w5056 _ _ _ _ _ _]
                  frame Default {
                    # "Do nothing ..."
                  }
                  frame 0 {
                    n1446 = case shown="72, 75, 77, 80" w5056 {
                      selector: w5056 -> [_ w5058]
                      frame Default {
                      }
                      frame 72, 75, 77, 80 {
                        # "Les 4 flèches ..."
                        # "Passer dans une astrométrie ?"
                        n1447 = local read "Servo"() -> (w5057:bool)
                        n1448 = case shown="Faux" w5057 {
                          tunnel: w5058 -> [w5072 _]
                          frame False {
                            # "Va marcher seulement 99.9% du temps, les SETs doivent être directement\nici si on veut éviter que ProcessedFalconImage ne puisse venir modifier\nles paramètres avant l'envoi."
                            n1449 = property on="ImgArray" class="GraphInt (strict)"("Active Cursor"=u32 0) -> (error out=w5069:errorcluster)  [unwired: 2 in, 1 out]
                            n1450 = property on="ImgArray" class="GraphInt (strict)"(error in=w5069) -> ("Cursor.Cursor X"=w5071:dbl, "Cursor.Cursor Y"=w5070:dbl)  [unwired: 1 in, 2 out]
                            n1451 = case shown="Par défaut" w5072 {
                              tunnel: w5071 -> [w5077 w5078 w5082 w5086 w5089]
                              tunnel: w5070 -> [w5076 w5080 w5083 w5085 w5087]
                              tunnel: [w5077 w5078 w5081 w5086 w5088] -> w5067
                              tunnel: [w5076 w5079 w5083 w5084 w5087] -> w5066
                              frame Default {
                              }
                              frame 72 {
                                # "\"Up\""
                                n1452 = Increment(x=w5080) -> (x+1=w5079:dbl)
                              }
                              frame 77 {
                                # "\"Right\""
                                n1453 = Increment(x=w5082) -> (x+1=w5081:dbl)
                              }
                              frame 80 {
                                # "\"Down\""
                                n1454 = Decrement(x=w5085) -> (x-1=w5084:dbl)
                              }
                              frame 75 {
                                # "\"Left\""
                                n1455 = Decrement(x=w5089) -> (x-1=w5088:dbl)
                              }
                            }
                            n1456 = local read "ROIWidth"() -> (w5065:u16)
                            n1457 = local read "ROIHeight"() -> (w5064:u16)
                            n1458 = control-ref of="ImgArray"() -> (w5059:refnum<vi>)
                            n1459 = call "SAOMM-Cursor2ROI.vi"("ImgRef"=w5059, "CursorX"=w5067, "CursorY"=w5066, "ROIWidth"=w5065, "ROIHeight"=w5064) -> ("XÉtoile"=w5060:dbl, "YÉtoile"=w5061:dbl, "ROIXOffset"=w5063:u16, "ROIYOffset"=w5062:u16)  [unwired: 7 in]
                            n1460 = local write "XReference"(w5060) -> ()
                            n1461 = local write "YReference"(w5061) -> ()
                            n1462 = flat-sequence {
                              tunnel: w5063 -> [w5074]
                              tunnel: w5062 -> [w5073]
                              frame #0 {
                                n1463 = local write "ROIXOffset"(w5074) -> ()
                                n1464 = local write "ROIYOffset"(w5073) -> ()
                              }
                              frame #1 {
                                n1465 = property on="UpdateROI" class="Bool (strict)"("Val(Sgnl)"=TRUE ("Value (Signaling)")) -> ()  [unwired: 2 in, 2 out]
                              }
                            }
                          }
                          frame True {
                            n1466 = One Button Dialog(message="Vous ne pouvez pas modifier la ROI pendant l'asservissement") -> ()  [unwired: 1 in, 1 out]
                          }
                        }
                      }
                    }
                  }
                  frame 9 {
                    # "tab"
                    n1467 = property on="Offset OK" class="Bool (strict)"() -> ("Key Focus"=w5091:bool)  [unwired: 2 in, 2 out]
                    n1468 = property on="N.O. A.D." class="Ch"() -> ("Key Focus"=w5095:bool)  [unwired: 2 in, 2 out]
                    n1469 = property on="N.O. Déc." class="Ch"() -> ("Key Focus"=w5096:bool)  [unwired: 2 in, 2 out]
                    n1470 = property on="NO epoch" class="NumNb (strict)"() -> ("Key Focus"=w5097:bool)  [unwired: 2 in, 2 out]
                    n1471 = property on="ModCoor" class="Bool (strict)"() -> ("Key Focus"=w5098:bool)  [unwired: 2 in, 2 out]
                    n1472 = property on="Offset RA" class="NumNb (strict)"() -> ("Key Focus"=w5093:bool)  [unwired: 2 in, 2 out]
                    n1473 = property on="Offset DEC" class="NumNb (strict)"() -> ("Key Focus"=w5092:bool)  [unwired: 2 in, 2 out]
                    n1474 = Compound Arithmetic op=OR(w5095, w5096, w5097, w5098, w5093, w5092, w5091) -> (w5094:bool)
                    n1475 = case shown="Faux" w5094 {
                      frame False {
                        n1476 = flat-sequence {
                          frame #0 {
                            n1477 = property on="N.O. A.D." class="Ch"("Key Focus"=TRUE) -> ()  [unwired: 2 in, 2 out]
                          }
                          frame #1 {
                            n1478 = property on="NO RA clic-sim" class="Bool (strict)"("Val(Sgnl)"=TRUE ("Value (Signaling)")) -> ()  [unwired: 2 in, 2 out]
                          }
                        }
                      }
                      frame True {
                      }
                    }
                  }
                  frame 32 {
                    # "Space bar"
                    n1479 = property on="Obslib" class="Tbl (strict)"() -> ("Key Focus"=w5101:bool)  [unwired: 2 in, 2 out]
                    n1480 = case shown="Faux" w5101 {
                      frame False {
                        n1481 = property on="Offset RA" class="NumNb (strict)"("Key Focus"=TRUE) -> ()  [unwired: 2 in, 2 out]
                      }
                      frame True {
                      }
                    }
                  }
                  frame 101 {
                    # "'e' pour Est"
                    n1482 = local read "Offset RA"() -> (w5104:dbl)
                    n1483 = Absolute Value(x=w5104) -> (abs(x)=w5103:dbl)
                    n1484 = property on="Offset RA" class="NumNb (strict)"("Val(Sgnl)"=w5103) -> ()  [unwired: 2 in, 2 out]
                  }
                  frame 110 {
                    # "'n' pour Nord"
                    n1485 = local read "Offset DEC"() -> (w5106:dbl)
                    n1486 = Absolute Value(x=w5106) -> (abs(x)=w5105:dbl)
                    n1487 = property on="Offset DEC" class="NumNb (strict)"("Val(Sgnl)"=w5105) -> ()  [unwired: 2 in, 2 out]
                  }
                  frame 111, 119 {
                    # "'o' ou 'w' pour Ouest"
                    n1488 = local read "Offset RA"() -> (w5109:dbl)
                    n1489 = Absolute Value(x=w5109) -> (abs(x)=w5108:dbl)
                    n1490 = Negate(x=w5108) -> (-x=w5107:dbl)
                    n1491 = property on="Offset RA" class="NumNb (strict)"("Val(Sgnl)"=w5107) -> ()  [unwired: 2 in, 2 out]
                  }
                  frame 115 {
                    # "'s' pour Sud"
                    n1492 = local read "Offset DEC"() -> (w5112:dbl)
                    n1493 = Absolute Value(x=w5112) -> (abs(x)=w5111:dbl)
                    n1494 = Negate(x=w5111) -> (-x=w5110:dbl)
                    n1495 = property on="Offset DEC" class="NumNb (strict)"("Val(Sgnl)"=w5110) -> ()  [unwired: 2 in, 2 out]
                  }
                }
              }
              event Mouse Move {
                n1496 = event-data() -> ()  [unwired: 1 in, 4 out]
                n1497 = disable-structure shown="Enabled" {
                  frame Disabled {
                    n1498 = while {
                      stop <- w5116 continue-if-true
                      w5117 = -1 ("x")
                      n1499 = property on="Picture" class="Image"() -> ("Mouse"=w5120:T39)  [unwired: 2 in, 2 out]
                      n1500 = Unbundle By Name(w5120) -> ("Mouse Position.X"=w5115:i32, "Mouse Position.Y"=w5114:i32, "Mouse Modifiers.Button Down"=w5113:bool)
                      n1501 = case shown="Vrai" w5113 {
                        frame False {
                        }
                        frame True {
                          n1502 = control-ref of="ImgArray"() -> (w5121:refnum<vi>)
                          n1503 = local write "Naxis1"(i16 640 ("Nx")) -> ()
                          n1504 = local write "Naxis2"(i16 480 ("Ny")) -> ()
                          n1505 = local write item#-1(i16 0 ("Xs")) -> ()
                          n1506 = local write item#-1(i16 0 ("Ys")) -> ()
                          n1507 = stacked-sequence {
                            seq-local: [w5127 _] -> [_ w5187]
                            seq-local: [w5126 _] -> [_ w5186]
                            tunnel: w5121 -> [w5128 _]
                            frame #0 {
                              n1508 = while {
                                tunnel: w5128 -> [w5131]
                                tunnel: [w5130] -> w5127
                                tunnel: [w5129] -> w5126
                                i -> [w5133]
                                stop <- w5132 continue-if-true
                                n1509 = property on="Picture" class="Image"() -> ("Mouse"=w5135:T39)  [unwired: 2 in, 2 out]
                                n1510 = Equal To 0?(x=w5133) -> (x = 0?=w5134:bool)
                                n1511 = Unbundle By Name(w5135) -> ("Mouse Position.X"=w5130:i32, "Mouse Position.Y"=w5129:i32, "Mouse Modifiers.Button Down"=w5132:bool)
                                n1512 = case shown="Faux" w5134 {
                                tunnel: w5130 -> [w5137 w5175]
                                tunnel: w5129 -> [w5136 w5156]
                                tunnel: w5131 -> [w5148 w5174]
                                frame False {
                                # "Correspond à la grandeur du picture pas de la caméra de guidage ..."
                                n1513 = local read item#-1() -> (w5153)
                                n1514 = local read item#-1() -> (w5154)
